vi "Complete Auth.vi"(8 "error in (no error)":errorcluster, 11 "Async Authorization in":refnum<class "Async Authorization.lvclass">) -> (0 "error out":errorcluster, 3 "Async Authorization out":refnum<class "Async Authorization.lvclass">)   [LabVIEW 2020, in "OAuth2.lvlib" / "Async Authorization.lvclass"]
uses:
  Async Authorization.lvclass
  Authorization/Authorization.lvclass
  Async Auth Result.ctl
  OAuth2.lvlib
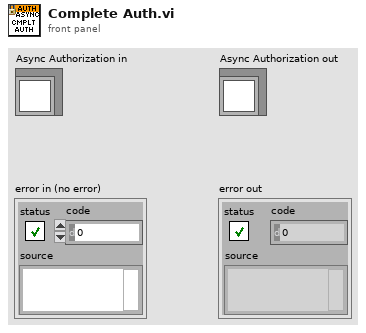
[diagram p1: front panel]
types:
  T1 = typedef "OAuth2.lvlib/Async Auth Result.ctl" = cluster{"Authorization":refnum<class "Authorization.lvclass">, "error":errorcluster}
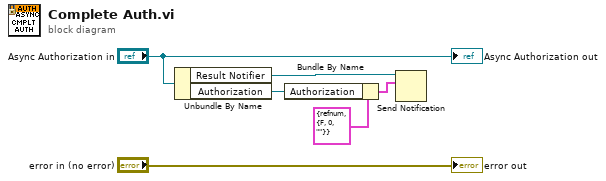
[diagram p0: block diagram]
diagram:
  n1 = Unbundle By Name("Async Authorization in") -> ("Result Notifier"=w4:refnum<notifier>, "Authorization"=w1:refnum<class "Authorization.lvclass">)
  n2 = Bundle By Name(cluster=T1 {"Authorization"=refnum, "error"={"status"=FALSE, "code"=0, "source"=""}} ("notification"), "Authorization"=w1) -> (w2:T1)
  n3 = Send Notification(notification=w2, notifier=w4) -> ()  [unwired: 1 in, 2 out]
  "error out" <- "error in (no error)"
  "Async Authorization out" <- "Async Authorization in"
